vi "Query Aperture Length.vi"(0 "VISA resource name":refnum<visa-resource-name>, 11 "error in (no error)":errorcluster) -> (4 "VISA resource name out":refnum<visa-resource-name>, 6 "Aperture Length (s)":dbl, 15 "error out":errorcluster)   [LabVIEW 2012, in "NH Research Regenerative Test Series.lvlib"]
doc: "Returns how long a measurement aperture is set to. The Module will pick the sample rate. The actual number of samples may be less than that specified in Set Max Samples.vi. Applies to both voltage and current measurements."
uses:
  <instrlib>/NH Research Regenerative Test Series/NH Research Regenerative Test Series.lvlib
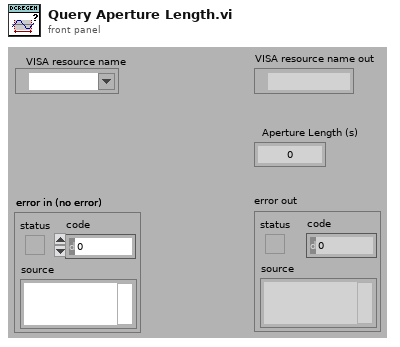
[diagram p1: front panel]
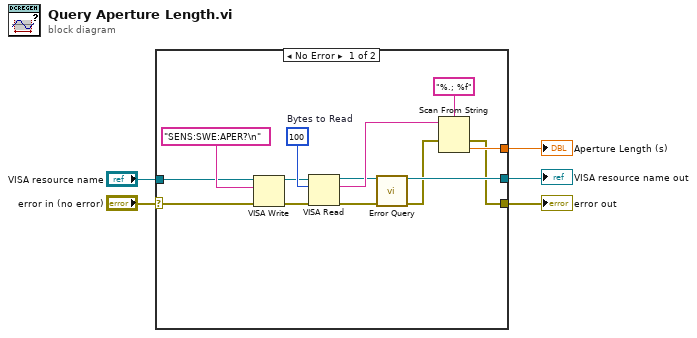
[diagram p0: block diagram]
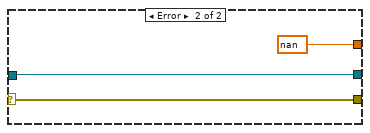
[diagram p2: hidden frame]
diagram:
  n1 = case shown="No Error" "error in (no error)" {
    selector: "error in (no error)" -> [w15 w22]
    tunnel: [w6 w22] -> w4
    tunnel: [w10 w21] -> w2
    tunnel: "VISA resource name" -> [w14 w21]
    tunnel: [w11 nan] -> w1
    frame No Error {
      w19 = u32 100  # Bytes to Read
      n2 = VISA Write(VISA resource name=w14, write buffer="SENS:SWE:APER?\n", error in (no error)=w15) -> (VISA resource name out=w17:refnum<visa-resource-name>, error out=w18:errorcluster)  [unwired: 1 out]
      n3 = VISA Read(VISA resource name=w17, byte count=w19, error in (no error)=w18) -> (VISA resource name out=w9:refnum<visa-resource-name>, read buffer=w13:string, error out=w8:errorcluster)  [unwired: 1 out]
      n4 = call <instrlib>:"Error Query.vi"("VISA resource name"=w9, "error in (no error)"=w8) -> ("VISA resource name out"=w10:refnum<visa-resource-name>, "error out"=w7:errorcluster)  [unwired: 10 in, 2 out]
      n5 = Scan From String(format string="%.; %f", input string=w13, error in=w7) -> (error out=w6:errorcluster, output 1=w11:dbl)  [unwired: 2 in, 2 out]
    }
    frame Error {
    }
  }
  "error out" <- w4
  "VISA resource name out" <- w2
  "Aperture Length (s)" <- w1
